vi "Get RX Message.vi"(8 "error in (no error)":errorcluster, 11 "RxTx in":refnum<class "RxTx.lvclass">) -> (0 "error out":errorcluster, 2 "new msg":bool, 3 "RxTx out":refnum<class "RxTx.lvclass">)   [LabVIEW 2018, in "RxTx.lvclass"]
doc: "Pop the lastest Rx message found in the qeue"
uses:
  RxTx.lvclass
  RxTx.lvclass/RxTx.ctl
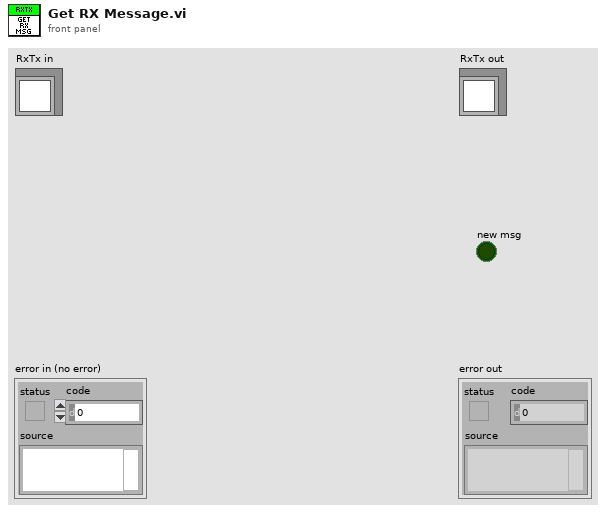
[diagram p1: front panel]
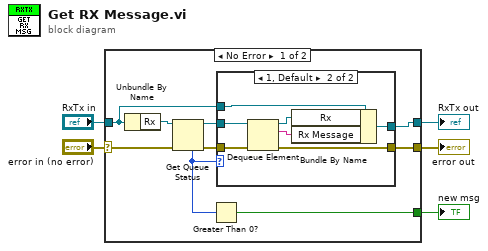
[diagram p0: block diagram]
diagram:
  n1 = case shown="No Error" "error in (no error)" {
    selector: "error in (no error)" -> [w11 w25]
    tunnel: [w9 w25] -> w2
    tunnel: [w13 w24] -> w3
    tunnel: "RxTx in" -> [w14 w24]
    tunnel: [w7 _] -> w1
    frame No Error {
      n2 = Unbundle By Name(w14) -> ("Rx"=w12:refnum<queue>)
      n3 = Get Queue Status(queue=w12, error in (no error)=w11) -> (queue out=w6:refnum<queue>, error out=w10:errorcluster, # elements in queue=w8:i32)  [unwired: 1 in, 5 out]
      n4 = Greater Than 0?(x=w8) -> (x > 0?=w7:bool)
      n5 = case shown="1, Default" w8 {
        tunnel: w6 -> [_ w23]
        tunnel: w14 -> [w15 w22]
        tunnel: [w15 w21] -> w13
        tunnel: w10 -> [w16 w19]
        tunnel: [w16 w18] -> w9
        frame 0 {
        }
        frame 1, Default {
          n6 = Dequeue Element(queue=w23, error in (no error)=w19) -> (queue out=w17:refnum<queue>, element=w20:string, error out=w18:errorcluster)  [unwired: 1 in, 1 out]
          n7 = Bundle By Name(cluster=w22, "Rx"=w17, "Rx Message"=w20) -> (w21:refnum<class "RxTx.lvclass">)
        }
      }
    }
    frame Error {
    }
  }
  "error out" <- w2
  "RxTx out" <- w3
  "new msg" <- w1
